vi "valve_colors_VCH.vi"(10 "Z_State":T2=enum."not ready", 11 "Z1(CmdSource)":T1(ring)) -> (0 "slide visible":bool, 1 "on visible":bool, 2 "auto visible":bool, 3 "N ring":u16)   [LabVIEW 2019, in "Valves.lvlib"]
uses:
  Valves.lvlib
  ctl/Z_State_VCH.ctl
  Trigers/D^.vi
  Logik/fronts.vi
  Timer Delay/Timer.vi
  Counter/Counter.lvlib
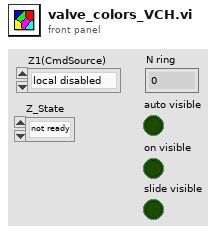
[diagram p1: front panel]
types:
  T1 = enum8{"local disabled", "local hand", "hand", "auto", "dist"}
  T2 = typedef "Valves.lvlib/Z_State_VCH.ctl" = enum8{"initialization", "alarm", "disabled", "not ready", "closed ready", "reserv", "reserv1", "reserv2", "reserv3", "check", "on min", "open", "on (closed)"}
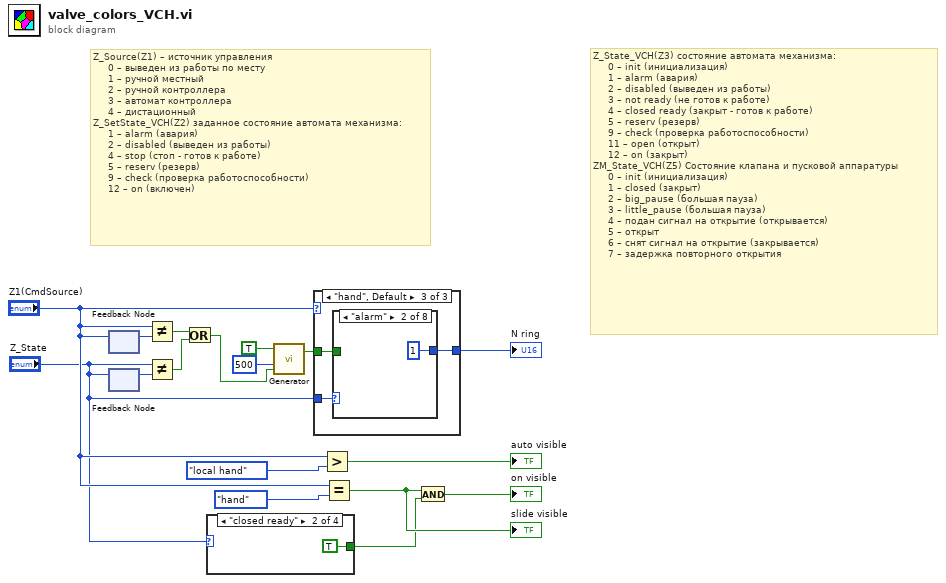
[diagram p0: block diagram]
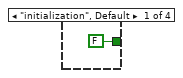
[diagram p2: hidden frame]
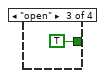
[diagram p3: hidden frame]
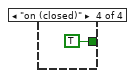
[diagram p4: hidden frame]
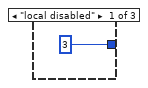
[diagram p5: hidden frame]
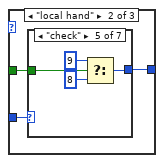
[diagram p6: hidden frame]
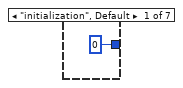
[diagram p7: hidden frame]
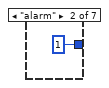
[diagram p8: hidden frame]
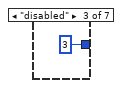
[diagram p9: hidden frame]
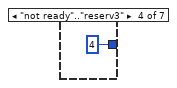
[diagram p10: hidden frame]
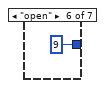
[diagram p11: hidden frame]
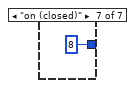
[diagram p12: hidden frame]
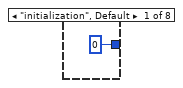
[diagram p13: hidden frame]
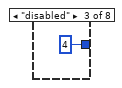
[diagram p14: hidden frame]
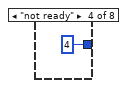
[diagram p15: hidden frame]
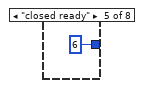
[diagram p16: hidden frame]
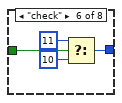
[diagram p17: hidden frame]
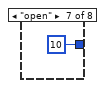
[diagram p18: hidden frame]
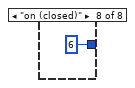
[diagram p19: hidden frame]
diagram:
  # "Z_State_VCH(Z3) состояние автомата механизма:\n     0 – init (инициализация)\n     1 – alarm (авария)\n     2 – disabled (выведен из работы)\n     3 – not ready (не готов к работе)\n     4 – closed ready (закрыт - готов к работе)\n     5 – reserv (резерв)\n     9 – check (проверка работоспособности)\n     11 – open (открыт)\n     12 – on (закрыт)\nZM_State_VCH(Z5) Состояние клапана и пусковой аппаратуры\n     0 – init (инициализация)\n     1 – сlosed (закрыт)\n     2 – big_pause (большая пауза)\n     3 – little_pause (большая пауза)\n     4 – подан сигнал на открытие (открывается)\n     5 – открыт\n     6 – снят сигнал на открытие (закрывается)\n     7 – задержка повторного открытия"
  # "Z_Source(Z1) – источник управления\n     0 – выведен из работы по месту\n     1 – ручной местный\n     2 – ручной контроллера\n     3 – автомат контроллера\n     4 – дистационный\nZ_SetState_VCH(Z2) заданное состояние автомата механизма:\n     1 – alarm (авария)\n     2 – disabled (выведен из работы)\n     4 – stop (стоп - готов к работе)\n     5 – reserv (резерв)\n     9 – check (проверка работоспособности)\n     12 – on (включен)"
  n1 = feedback #1() -> (w14:T1)  [unwired: 1 in]
  n2 = feedback-in #1("Z1(CmdSource)") -> ()
  n3 = feedback #2() -> (w13:T2)  [unwired: 1 in]
  n4 = feedback-in #2("Z_State") -> ()
  n5 = Not Equal?(x="Z1(CmdSource)", y=w14) -> (x != y?=w12:bool)
  n6 = Not Equal?(x="Z_State", y=w13) -> (x != y?=w11:bool)
  n7 = Or(x=w12, y=w11) -> (x .or. y?=w10:bool)
  n8 = case shown="\"closed ready\"" "Z_State" {
    tunnel: [FALSE TRUE TRUE TRUE] -> w1
    frame "initialization", Default {
    }
    frame "closed ready" {
    }
    frame "open" {
    }
    frame "on (closed)" {
    }
  }
  n9 = call "Generator.vi"("R"=w10, "T ms (500)"=u32 500 ("T (ms)"), "ON (F)"=TRUE ("ON")) -> ("Q"=w15:bool)  [unwired: 1 in]
  n10 = case shown="\"hand\", Default" "Z1(CmdSource)" {
    tunnel: w15 -> [_ w25 w37]
    tunnel: "Z_State" -> [_ w24 w38]
    tunnel: [u16 3 ("Z5 ind") w23 w36] -> w9
    frame "local disabled" {
    }
    frame "local hand" {
      n11 = case shown="\"check\"" w24 {
        tunnel: [u16 0 ("Z5 ind") u16 1 ("Z5 ind") u16 3 ("Z5 ind") u16 4 ("Z5 ind") w31 u16 9 ("Z5 ind") u16 8 ("Z5 ind")] -> w23
        tunnel: w25 -> [_ _ _ _ w30 _ _]
        frame "initialization", Default {
        }
        frame "alarm" {
        }
        frame "disabled" {
        }
        frame "not ready".."reserv3" {
        }
        frame "check" {
          n12 = Select(t=u16 9 ("Z5 ind"), s=w30, f=u16 8) -> (s? t:f=w31:u16)
        }
        frame "open" {
        }
        frame "on (closed)" {
        }
      }
    }
    frame "hand", Default {
      n13 = case shown="\"alarm\"" w38 {
        tunnel: [u16 0 ("Z5 ind") u16 1 ("Z5 ind") u16 4 ("Z5 ind") u16 4 ("Z5 ind") u16 6 ("Z5 ind") w45 u16 10 ("Z5 ind") u16 6 ("Z5 ind")] -> w36
        tunnel: w37 -> [_ _ _ _ _ w44 _ _]
        frame "initialization", Default {
        }
        frame "alarm" {
        }
        frame "disabled" {
        }
        frame "not ready" {
        }
        frame "closed ready" {
        }
        frame "check" {
          n14 = Select(t=u16 11 ("Z5 ind"), s=w44, f=u16 10) -> (s? t:f=w45:u16)
        }
        frame "open" {
        }
        frame "on (closed)" {
        }
      }
    }
  }
  "N ring" <- w9
  n15 = Greater?(x="Z1(CmdSource)", y=T1."local hand" ("Z1(CmdSource) 2")) -> (0:→"auto visible":bool)
  n16 = Equal?(x="Z1(CmdSource)", y=T1."hand" ("Z1(CmdSource) 2")) -> (x = y?=w6:bool)
  "slide visible" <- w6
  n17 = And(x=w6, y=w1) -> (x .and. y?=→"on visible":bool)
